vi "convert.vi"(11 "point":cluster{"x":dbl, "y":dbl}) -> (3 "scaled":cluster{"x":dbl, "y":dbl})   [LabVIEW 2022 SP3]
uses:
  Perspective_Globals.vi
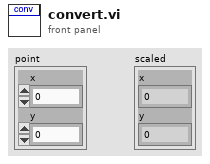
[diagram p1: front panel]
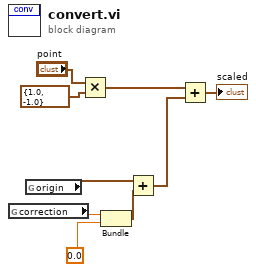
[diagram p0: block diagram]
diagram:
  n1 = global read "Perspective_Globals.vi" "correction"() -> (w2:dbl)
  n2 = global read "Perspective_Globals.vi" "origin"() -> (w4:cluster{"x":dbl, "y":dbl})
  n3 = Multiply(x="point", y=cluster{"x":dbl, "y":dbl} {"x"=1.0, "y"=-1.0} ("origin")) -> (x*y=w7:cluster{"x":dbl, "y":dbl})
  n4 = Bundle("correction"=w2, "x"=0.0) -> (w5:cluster{"correction":dbl, "x":dbl})  [unwired: 1 in]
  n5 = Add(x=w4, y=w5) -> (x+y=w3:cluster{dbl, dbl})
  n6 = Add(x=w7, y=w3) -> (x+y=→"scaled":cluster{dbl, dbl})
